vi "Slave2.vi"() -> ()   [LabVIEW 2012]
uses:
  MyGlobals.vi
panel:
  out "Slave2Text":string
  in  "Slave2 Original":string="Name "
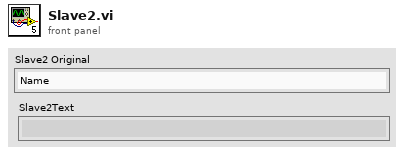
[diagram p1: front panel]
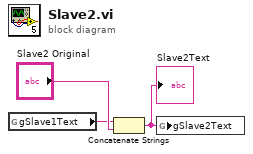
[diagram p0: block diagram]
diagram:
  n1 = global read "MyGlobals.vi" "gSlave1Text"() -> (w1:string)
  n2 = Concatenate Strings(w1, "Slave2 Original") -> (w2:string)
  "Slave2Text" <- w2
  n3 = global write "MyGlobals.vi" "gSlave2Text"(w2) -> ()
